vi "sub_DTMF Tone.vi"(8 "error in (no error)":errorcluster, 11 "Key Character":string) -> (0 "error out":errorcluster, 1 "Low Frequency":dbl, 3 "High Frequency":dbl)   [LabVIEW 2014]
doc: "------------------------------------\nAuther: Koji Ohashi\nCopyright (c) 2020 Japan LabVIEW Users Group, Volunteer members.\nThis VI is released under the MIT License.\nhttp://opensource.org/licenses/mit-license.php\n------------------------------------"
panel:
  out "floor(x/y)":i32
  out "x-y*floor(x/y)":i32
  out "index of element":i32
  out "1D array":string[](array[string])
  out "1stCharacter":string
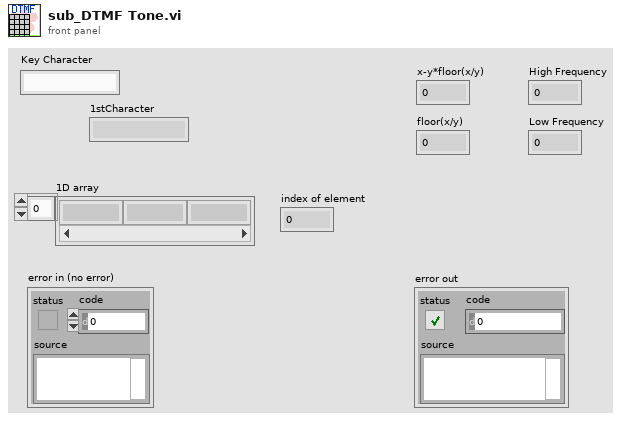
[diagram p1: front panel]
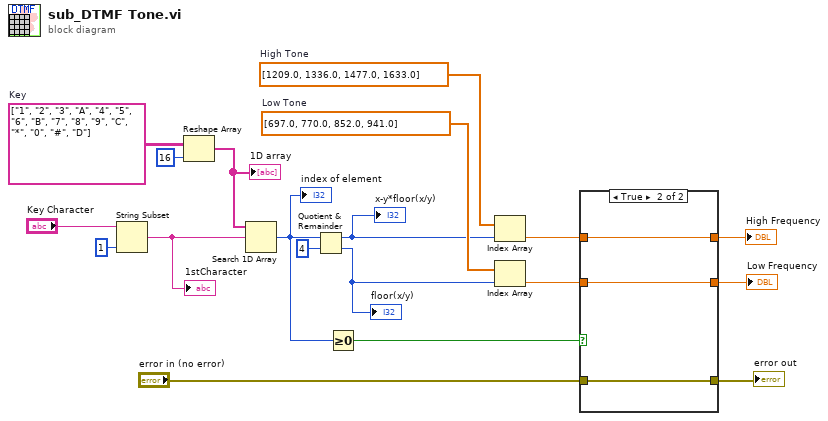
[diagram p0: block diagram]
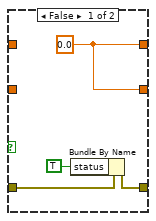
[diagram p2: hidden frame]
diagram:
  w11 = dbl[] [1209.0, 1336.0, 1477.0, 1633.0]  # High Tone
  w12 = dbl[] [697.0, 770.0, 852.0, 941.0]  # Low Tone
  w17 = string[][] [["1", "2", "3", "A"], ["4", "5", "6", "B"], ["7", "8", "9", "C"], ["*", "0", "#", "D"]]  # Key
  n1 = String Subset(string="Key Character", length (rest)=1 ("length (rest)")) -> (substring=w14:string)  [unwired: 1 in]
  "1stCharacter" <- w14
  n2 = Reshape Array "Reshape Array"(w17, 16 ("dimension size")) -> (w15:string[])
  "1D array" <- w15
  n3 = Search 1D Array(1D array=w15, element=w14) -> (index of element=w8:i32)  [unwired: 1 in]
  "index of element" <- w8
  n4 = Quotient & Remainder(x=w8, y=4) -> (x-y*floor(x/y)=w10:i32, floor(x/y)=w9:i32)
  "x-y*floor(x/y)" <- w10
  "floor(x/y)" <- w9
  n5 = Greater Or Equal To 0?(x=w8) -> (x >= 0?=w7:bool)
  n6 = Index Array "Index Array"(array=w11, index=w10) -> (element=w4:dbl)
  n7 = Index Array "Index Array"(array=w12, index=w9) -> (element=w3:dbl)
  n8 = case shown="TRUE" w7 {
    tunnel: [w22 w26] -> w5
    tunnel: "error in (no error)" -> [w23 w26]
    tunnel: [w20 w25] -> w2
    tunnel: w4 -> [_ w25]
    tunnel: [w20 w24] -> w1
    tunnel: w3 -> [_ w24]
    frame False {
      w20 = 0.0
      n9 = Bundle By Name(cluster=w23, "status"=TRUE) -> (w22:errorcluster)
    }
    frame True {
    }
  }
  "High Frequency" <- w2
  "Low Frequency" <- w1
  "error out" <- w5
